vi "Editor.vi"(9 "Editor Events":T15, 11 "Printer Settings In":refnum<class "Printer Settings.lvclass">) -> (3 "Printer Settings Out":refnum<class "Printer Settings.lvclass">)   [LabVIEW 2023, in "VIDoc Printer.lvlib" / "Printer Settings.lvclass"]
uses:
  Printer Settings.lvclass
  Editors/VIDoc Editor/Editor Events Cluster.ctl
  Project Settings.ctl
  Interface Settings.ctl
  Detail Level Enum.ctl
  Scope Settings.ctl
  Class Settings.ctl
  Library Settings.ctl
  VI Settings.ctl
  Control Settings.ctl
  LLB Settings.ctl
  Formatting Options.ctl
  Background Formatting Cluster.ctl
  Bookmark Options.ctl
  Printer Settings.lvclass/Printer Settings.ctl
  Editors/VIDoc Editor/VIDocEditor.lvclass
panel:
  in  "Sections Tabs":T1(tab)
  in  "Format Options":T2={"Background"={"Public Scope"={"Option"=FALSE, "Color"=0, "Operator"=FALSE}, "Protected Scope"={"Option"=FALSE, "Color"=0, "Operator"=FALSE}, "Community Scope"={"Option"=FALSE, "Color"=0, "Operator"=FALSE}, "Private Scope"={"Option"=FALSE, "Color"=0, "Operator"=FALSE}, "Unknown Scope"={"Option"=FALSE, "Color"=0, "Operator"=FALSE}, "Auto Error Handling"={"Option"=FALSE, "Color"=0, "Operator"=FALSE}, "Inline"={"Option"=FALSE, "Color"=0, "Operator"=FALSE}, "Separate CC"={"Option"=FALSE, "Color"=0, "Operator"=FALSE}, "Execution Priority Normal"={"Option"=FALSE, "Color"=0, "Operator"=FALSE}, "Reentrancy Non-RE"={"Option"=FALSE, "Color"=0, "Operator"=FALSE}}, "Bookmark Options"={"Bookmarks as New Line in VI Descriptions"=TRUE, "Unique Bookmark Tags Only"=TRUE, "Include Tag and Text"=TRUE}}
  in  "Library Scope":T5={"Public"=TRUE, "Community"=TRUE, "Private"=TRUE, "Unknown"=TRUE}
  in  "Projects Enabled":bool=TRUE caption="Enabled"
  in  "Project":T6={"Paths"=TRUE, "Descriptions"=TRUE, "Memory"=TRUE, "Options"=TRUE, "Symbols"=TRUE}
  in  "Bookmark Term Settings":cluster{"Term":string, "Settings":T7}[](array[cluster])
  in  "Interface":T9={"Memory"=TRUE, "By List"=TRUE, "Details"=TRUE, "Detail Options"={"Description"=TRUE, "Properties"=TRUE, "Inheritance"=TRUE, "Inheritance Options"={"Parent Interfaces"=TRUE, "Friends"=TRUE}}, "List Detail Level"=enum."None", "Controls Detail Level"=enum."None", "Methods Detail Level"=enum."None", "Controls Scope"={"Public"=TRUE, "Protected"=TRUE, "Community"=TRUE, "Private"=TRUE, "Unknown"=TRUE}, "Methods Scope"={"Public"=TRUE, "Protected"=TRUE, "Community"=TRUE, "Private"=TRUE, "Unknown"=TRUE}}
  in  "Interfaces Enabled":bool=TRUE caption="Enabled"
  in  "Class":T11={"Memory"=TRUE, "By Folder"=TRUE, "By Tree"=TRUE, "By List"=TRUE, "Details"=TRUE, "Detail Options"={"Description"=TRUE, "Properties"=TRUE, "Inheritance"=TRUE, "Inheritance Options"={"Parent Classes"=TRUE, "Parent Interfaces"=TRUE, "Parent Libraries"=TRUE, "Friends"=TRUE}}, "CPD Detail Level"=enum."None", "List Detail Level"=enum."None", "Controls Detail Level"=enum."None", "Methods Detail Level"=enum."None", "Set Accessor Detail Level"=enum."None", "Get Accessor Detail Level"=enum."None", "Controls Scope"={"Public"=TRUE, "Protected"=TRUE, "Community"=TRUE, "Private"=TRUE, "Unknown"=TRUE}, "Methods Scope"={"Public"=TRUE, "Protected"=TRUE, "Community"=TRUE, "Private"=TRUE, "Unknown"=TRUE}, "Get Accessors Scope"={"Public"=TRUE, "Protected"=TRUE, "Community"=TRUE, "Private"=TRUE, "Unknown"=TRUE}, "Set Accessors Scope"={"Public"=TRUE, "Protected"=TRUE, "Community"=TRUE, "Private"=TRUE, "Unknown"=TRUE}}
  in  "Classes Enabled":bool=TRUE caption="Enabled"
  in  "Library":T12={"Memory"=TRUE, "By Folder"=TRUE, "By Tree"=TRUE, "By List"=TRUE, "Details"=TRUE, "Detail Options"={"Description"=TRUE, "Properties"=TRUE, "Friends"=TRUE, "Child Libraries"=TRUE}, "List Detail Level"=enum."None", "Methods Detail Level"=enum."None", "Controls Detail Level"=enum."None", "Methods Scope"={"Public"=TRUE, "Protected"=TRUE, "Community"=TRUE, "Private"=TRUE, "Unknown"=TRUE}, "Controls Scope"={"Public"=TRUE, "Protected"=TRUE, "Community"=TRUE, "Private"=TRUE, "Unknown"=TRUE}}
  in  "Libraries Enabled":bool=TRUE caption="Enabled"
  in  "VI Member":T7={"Memory"=TRUE, "By Folder"=TRUE, "By Tree"=TRUE, "By List"=TRUE, "Methods"=TRUE, "Method Options"={"Front Panels"=TRUE, "Options"=TRUE, "Controls"=TRUE}, "List Detail Level"=enum."None", "Methods Detail Level"=enum."None", "Controls Detail Level"=enum."None"}
  in  "VI Methods Enabled":bool=TRUE caption="Enabled"
  in  "Control Member":T13={"Memory"=TRUE, "By Folder"=TRUE, "By Tree"=TRUE, "By List"=TRUE, "Controls"=TRUE, "List Detail Level"=enum."None", "Controls Detail Level"=enum."None"}
  in  "Control Methods Enabled":bool=TRUE caption="Enabled"
  in  "LLB":T14={"Methods"=TRUE, "Controls"=TRUE, "Methods Detail Level"=enum."None", "Controls Detail Level"=enum."None"}
  in  "LLBs Enabled":bool=TRUE caption="Enabled"
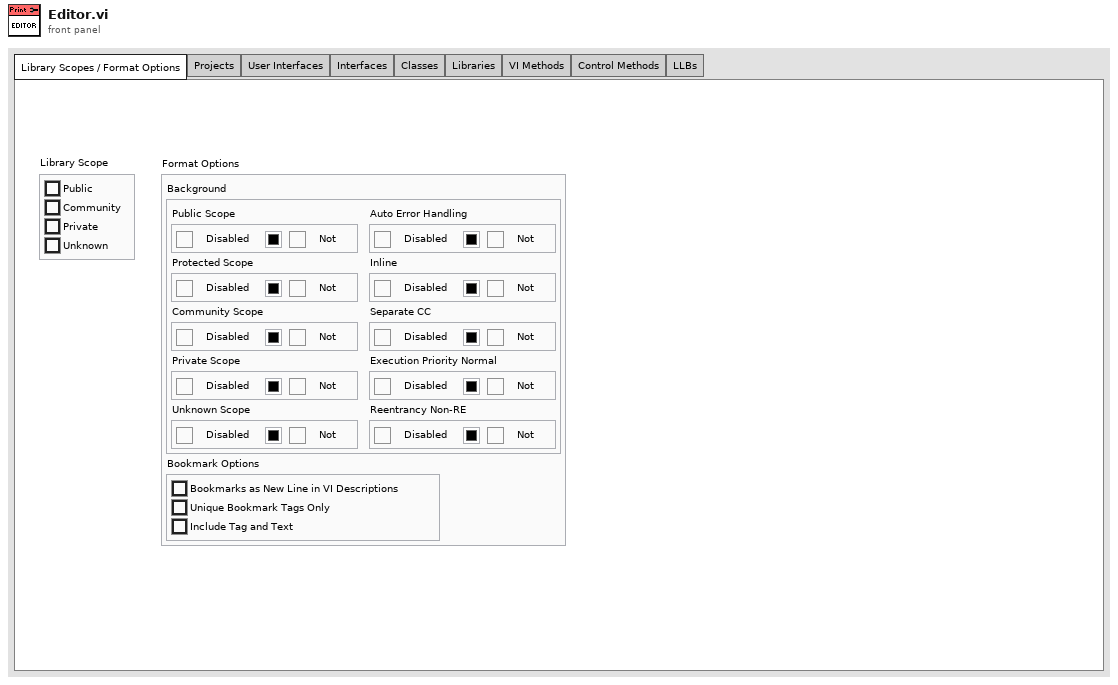
[diagram p1: front panel]
types:
  T1 = enum32{"Library Scopes / Format Options", "Projects", "User Interfaces", "Interfaces", "Classes", "Libraries", "VI Methods", "Control Methods", "LLBs"}
  T2 = typedef "VIDoc Printer.lvlib/Printer Settings.lvclass/Formatting Options.ctl" = cluster{"Background":cluster{"Public Scope":T3, "Protected Scope":T3, "Community Scope":T3, "Private Scope":T3, "Unknown Scope":T3, "Auto Error Handling":T3, "Inline":T3, "Separate CC":T3, "Execution Priority Normal":T3, "Reentrancy Non-RE":T3}, "Bookmark Options":T4}
  T3 = typedef "VIDoc Printer.lvlib/Printer Settings.lvclass/Background Formatting Cluster.ctl" = cluster{"Option":bool, "Color":u32, "Operator":bool}
  T4 = typedef "VIDoc Printer.lvlib/Printer Settings.lvclass/Bookmark Options.ctl" = cluster{"Bookmarks as New Line in VI Descriptions":bool, "Unique Bookmark Tags Only":bool, "Include Tag and Text":bool}
  T5 = cluster{"Public":bool, "Community":bool, "Private":bool, "Unknown":bool}
  T6 = typedef "VIDoc Printer.lvlib/Printer Settings.lvclass/Project Settings.ctl" = cluster{"Paths":bool, "Descriptions":bool, "Memory":bool, "Options":bool, "Symbols":bool}
  T7 = typedef "VIDoc Printer.lvlib/Printer Settings.lvclass/VI Settings.ctl" = cluster{"Memory":bool, "By Folder":bool, "By Tree":bool, "By List":bool, "Methods":bool, "Method Options":cluster{"Front Panels":bool, "Options":bool, "Controls":bool}, "List Detail Level":T8, "Methods Detail Level":T8, "Controls Detail Level":T8}
  T8 = typedef "VIDoc Printer.lvlib/Printer Settings.lvclass/Detail Level Enum.ctl" = enum16{"None", "Minimal", "Standard", "Full"}
  T9 = typedef "VIDoc Printer.lvlib/Printer Settings.lvclass/Interface Settings.ctl" = cluster{"Memory":bool, "By List":bool, "Details":bool, "Detail Options":cluster{"Description":bool, "Properties":bool, "Inheritance":bool, "Inheritance Options":cluster{"Parent Interfaces":bool, "Friends":bool}}, "List Detail Level":T8, "Controls Detail Level":T8, "Methods Detail Level":T8, "Controls Scope":T10, "Methods Scope":T10}
  T10 = typedef "VIDoc Printer.lvlib/Printer Settings.lvclass/Scope Settings.ctl" = cluster{"Public":bool, "Protected":bool, "Community":bool, "Private":bool, "Unknown":bool}
  T11 = typedef "VIDoc Printer.lvlib/Printer Settings.lvclass/Class Settings.ctl" = cluster{"Memory":bool, "By Folder":bool, "By Tree":bool, "By List":bool, "Details":bool, "Detail Options":cluster{"Description":bool, "Properties":bool, "Inheritance":bool, "Inheritance Options":cluster{"Parent Classes":bool, "Parent Interfaces":bool, "Parent Libraries":bool, "Friends":bool}}, "CPD Detail Level":T8, "List Detail Level":T8, "Controls Detail Level":T8, "Methods Detail Level":T8, "Set Accessor Detail Level":T8, "Get Accessor Detail Level":T8, "Controls Scope":T10, "Methods Scope":T10, "Get Accessors Scope":T10, "Set Accessors Scope":T10}
  T12 = typedef "VIDoc Printer.lvlib/Printer Settings.lvclass/Library Settings.ctl" = cluster{"Memory":bool, "By Folder":bool, "By Tree":bool, "By List":bool, "Details":bool, "Detail Options":cluster{"Description":bool, "Properties":bool, "Friends":bool, "Child Libraries":bool}, "List Detail Level":T8, "Methods Detail Level":T8, "Controls Detail Level":T8, "Methods Scope":T10, "Controls Scope":T10}
  T13 = typedef "VIDoc Printer.lvlib/Printer Settings.lvclass/Control Settings.ctl" = cluster{"Memory":bool, "By Folder":bool, "By Tree":bool, "By List":bool, "Controls":bool, "List Detail Level":T8, "Controls Detail Level":T8}
  T14 = typedef "VIDoc Printer.lvlib/Printer Settings.lvclass/LLB Settings.ctl" = cluster{"Methods":bool, "Controls":bool, "Methods Detail Level":T8, "Controls Detail Level":T8}
  T15 = typedef "VIDocEditor.lvclass/Editor Events Cluster.ctl" = cluster{"Close":refnum<user-event>, "Revert":refnum<user-event>, "Save":refnum<user-event>, "Changes?":refnum<user-event>}
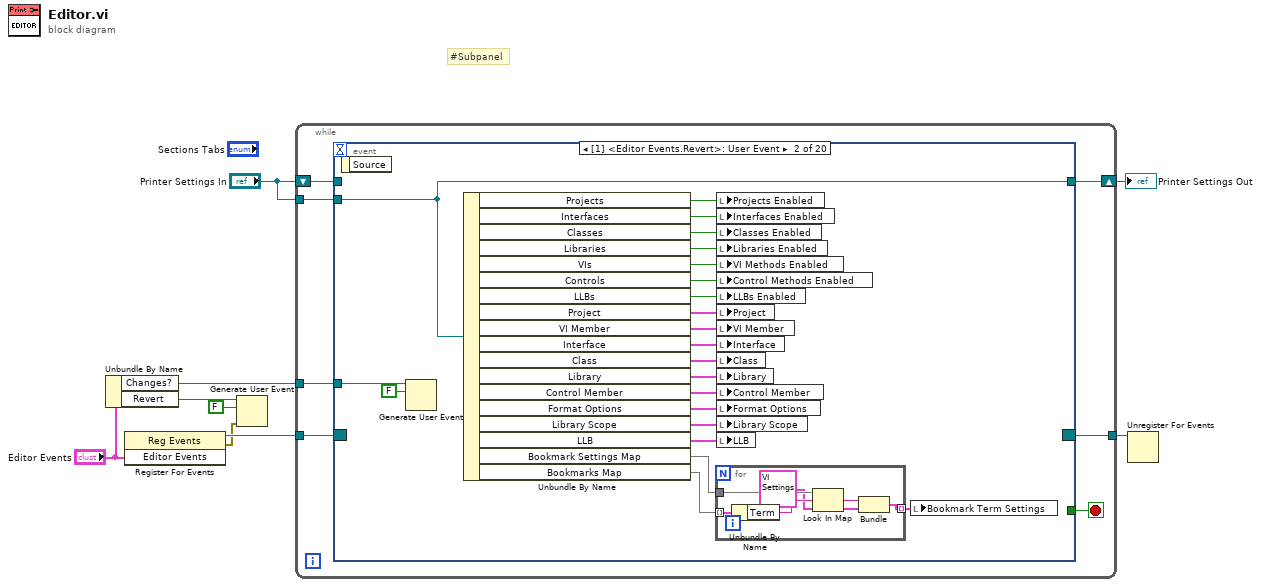
[diagram p0: block diagram]
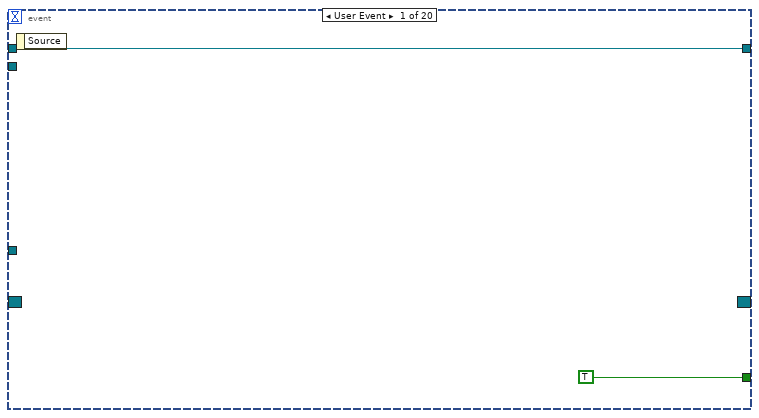
[diagram p2: hidden frame]
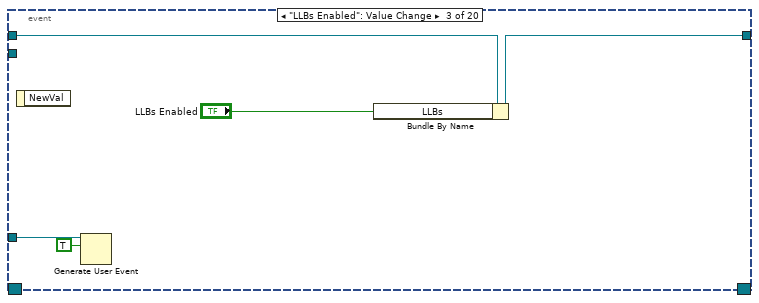
[diagram p3: hidden frame]
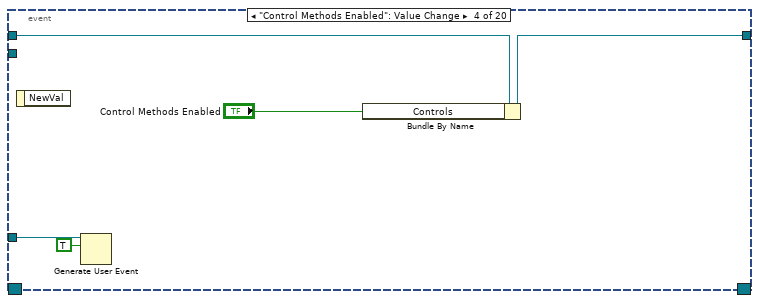
[diagram p4: hidden frame]
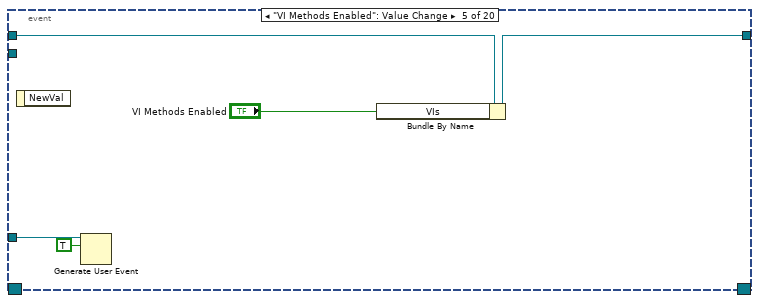
[diagram p5: hidden frame]
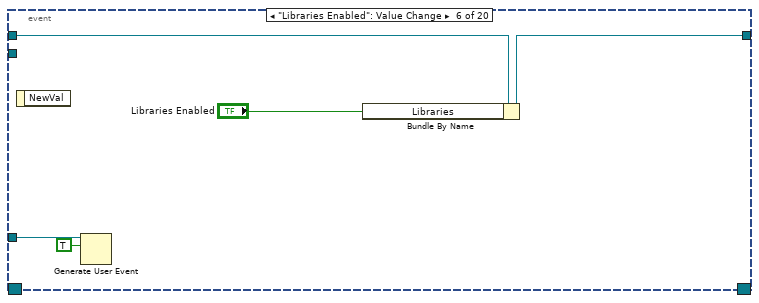
[diagram p6: hidden frame]
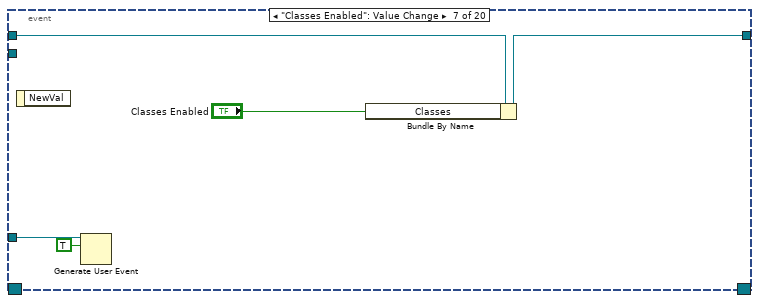
[diagram p7: hidden frame]
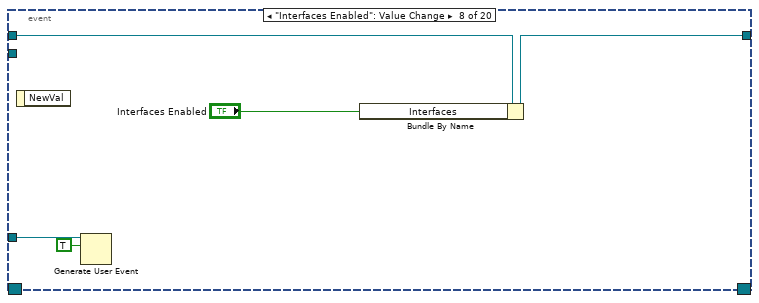
[diagram p8: hidden frame]
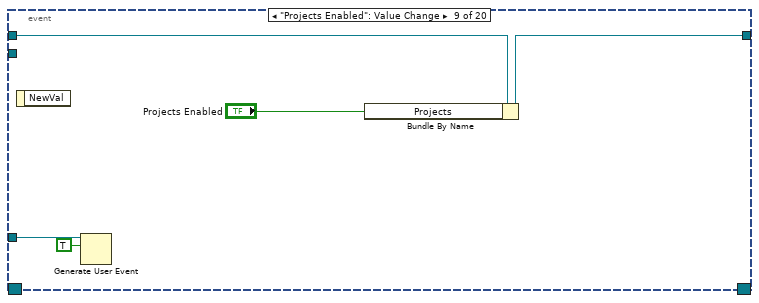
[diagram p9: hidden frame]
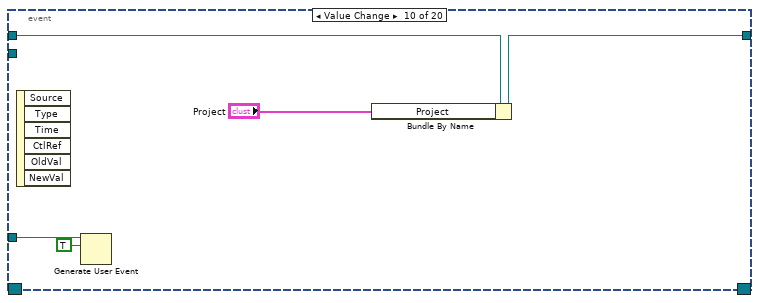
[diagram p10: hidden frame]
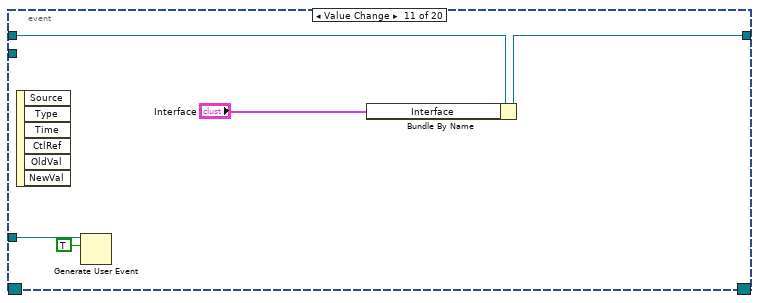
[diagram p11: hidden frame]
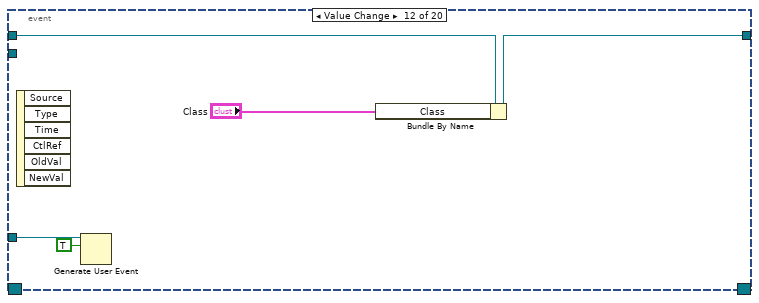
[diagram p12: hidden frame]
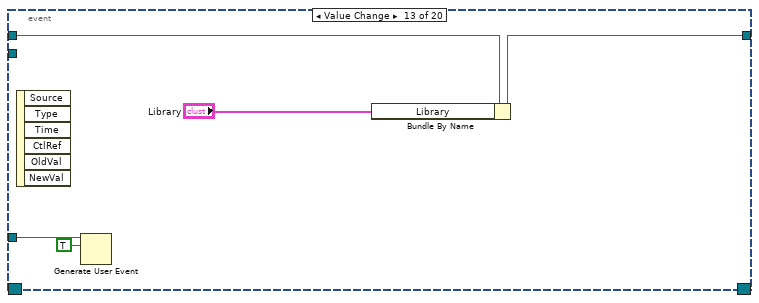
[diagram p13: hidden frame]
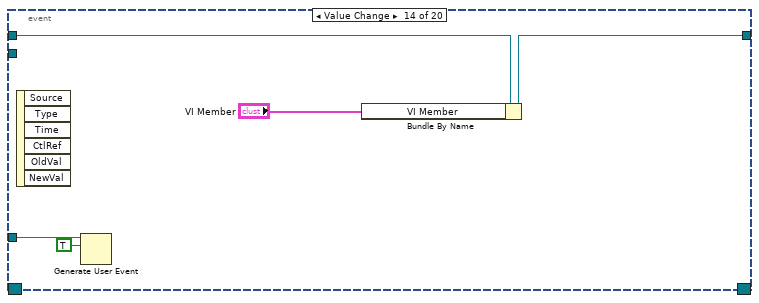
[diagram p14: hidden frame]
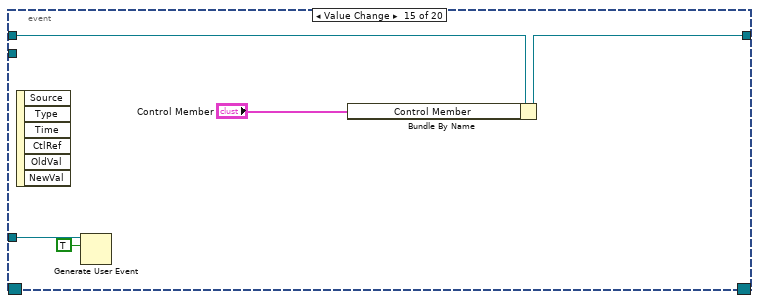
[diagram p15: hidden frame]
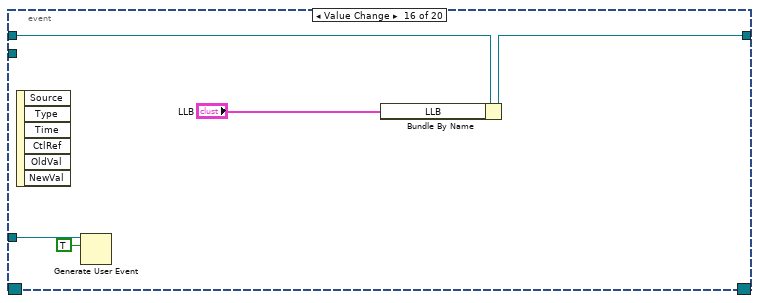
[diagram p16: hidden frame]
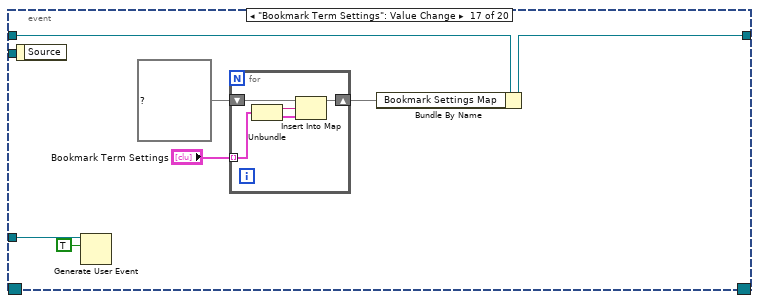
[diagram p17: hidden frame]
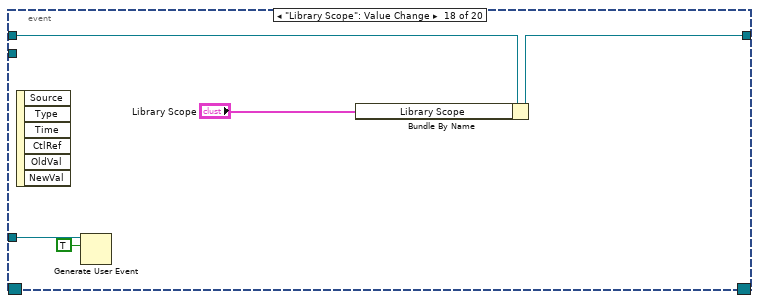
[diagram p18: hidden frame]
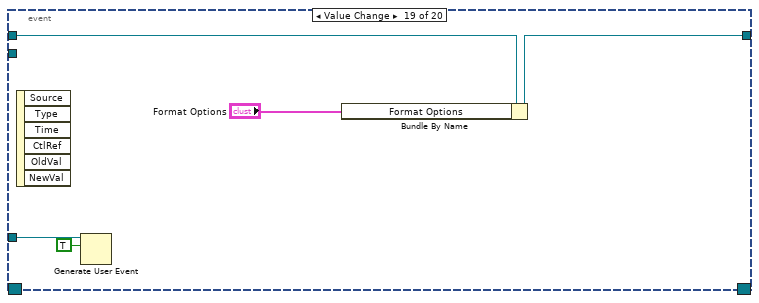
[diagram p19: hidden frame]
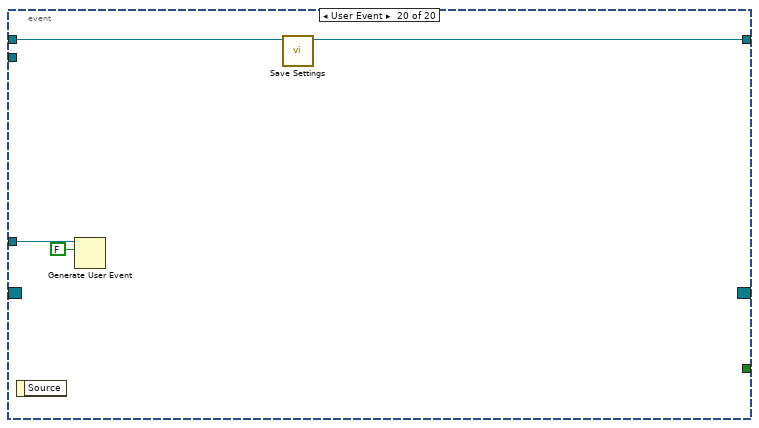
[diagram p20: hidden frame]
diagram:
  # "#Subpanel"
  n1 = Unbundle By Name("Editor Events") -> ("Changes?"=w1:refnum<user-event>, "Revert"=w4:refnum<user-event>)
  n2 = register-events("Editor Events") -> (reference out=w9:refnum<event-registration>, error out=w2:errorcluster)  [unwired: 2 in]
  n3 = Generate User Event(user event=w4, event data cluster=FALSE ("event data"), error in=w2) -> ()  [unwired: 1 in, 2 out]
  n4 = while {
    shift-right: [w14] -> w7
    shift-left: "Printer Settings In" -> [w16]
    tunnel: w9 -> [w15]
    tunnel: [w12] -> w8
    tunnel: "Printer Settings In" -> [w11]
    tunnel: w1 -> [w10]
    stop <- w13 stop-if-true
    n5 = event shown="[1] <Editor Events.Revert>: User Event" {
      selector: w15 -> [_ _ _ _ _ _ _ _ _ _ _ _ _ _ _ _ _ _ _ _]
      dyn-events: [_ _ _ _ _ _ _ _ _ _ _ _ _ _ _ _ _ _ _ _] -> w12
      timeout: _ -> [_ _ _ _ _ _ _ _ _ _ _ _ _ _ _ _ _ _ _ _]
      tunnel: w16 -> [w18 _ w51 w56 w61 w66 w71 w76 w81 w86 w91 w96 w101 w106 w111 w116 w123 w133 w138 w141]
      tunnel: [w18 w40 w50 w55 w60 w65 w70 w75 w80 w85 w90 w95 w100 w105 w110 w115 w122 w132 w137 w142] -> w14
      tunnel: [TRUE _ _ _ _ _ _ _ _ _ _ _ _ _ _ _ _ _ _ _] -> w13
      tunnel: w11 -> [_ w40 _ _ _ _ _ _ _ _ _ _ _ _ _ _ _ _ _ _]
      tunnel: w10 -> [_ w38 w47 w53 w58 w63 w68 w73 w78 w83 w88 w93 w98 w103 w108 w113 w120 w130 w135 w139]
      event User Event {
        n6 = event-data() -> ()  [unwired: 1 in, 1 out]
      }
      event User Event {
        n7 = event-data() -> ()  [unwired: 1 in, 1 out]
        n8 = Generate User Event(user event=w38, event data cluster=FALSE ("event data")) -> ()  [unwired: 2 in, 2 out]
        n9 = Unbundle By Name(w40) -> ("Projects"=w37:bool, "Interfaces"=w36:bool, "Classes"=w35:bool, "Libraries"=w34:bool, "VIs"=w33:bool, "Controls"=w32:bool, "LLBs"=w31:bool, "Project"=w29:T6, "VI Member"=w28:T7, "Interface"=w27:T9, "Class"=w26:T11, "Library"=w25:T12, "Control Member"=w24:T13, "Format Options"=w23:T2, "Library Scope"=w22:T5, "LLB"=w30:T14, "Bookmark Settings Map"=w20:map{string, T7}, "Bookmarks Map"=w21:map{string, string[]})
        n10 = for {
          tunnel: w21 -> [w46] mode=indexing
          tunnel: w20 -> [w45]
          tunnel: [w42] -> w19 mode=indexing
          n11 = Unbundle By Name(w46) -> ("Term"=w43:string)
          n12 = Look In Map(map=w45, key=w43, default value=T7 {"Memory"=FALSE, "By Folder"=FALSE, "By Tree"=TRUE, "By List"=FALSE, "Methods"=FALSE, "Method Options"={"Front Panels"=FALSE, "Options"=FALSE, "Controls"=FALSE}, "List Detail Level"=enum."Minimal", "Methods Detail Level"=enum."Minimal", "Controls Detail Level"=enum."Minimal"}) -> (value=w44:T7)  [unwired: 1 out]
          n13 = Bundle("Term"=w43, "Term Settings"=w44) -> (w42:cluster{"Term":string, "Term Settings":T7})  [unwired: 1 in]
        }
        n14 = local write "Projects Enabled"(w37) -> ()
        n15 = local write "Interfaces Enabled"(w36) -> ()
        n16 = local write "Classes Enabled"(w35) -> ()
        n17 = local write "Libraries Enabled"(w34) -> ()
        n18 = local write "VI Methods Enabled"(w33) -> ()
        n19 = local write "Control Methods Enabled"(w32) -> ()
        n20 = local write "LLBs Enabled"(w31) -> ()
        n21 = local write "Project"(w29) -> ()
        n22 = local write "VI Member"(w28) -> ()
        n23 = local write "Interface"(w27) -> ()
        n24 = local write "Class"(w26) -> ()
        n25 = local write "Library"(w25) -> ()
        n26 = local write "Control Member"(w24) -> ()
        n27 = local write "Format Options"(w23) -> ()
        n28 = local write "Library Scope"(w22) -> ()
        n29 = local write "LLB"(w30) -> ()
        n30 = local write "Bookmark Term Settings"(w19) -> ()
      }
      event "LLBs Enabled": Value Change {
        n31 = event-data() -> ()  [unwired: 1 in, 1 out]
        n32 = Generate User Event(user event=w47, event data cluster=TRUE ("event data")) -> ()  [unwired: 2 in, 2 out]
        n33 = Bundle By Name(cluster=w51, "LLBs"="LLBs Enabled") -> (w50:refnum<class "Printer Settings.lvclass">)
      }
      event "Control Methods Enabled": Value Change {
        n34 = event-data() -> ()  [unwired: 1 in, 1 out]
        n35 = Generate User Event(user event=w53, event data cluster=TRUE ("event data")) -> ()  [unwired: 2 in, 2 out]
        n36 = Bundle By Name(cluster=w56, "Controls"="Control Methods Enabled") -> (w55:refnum<class "Printer Settings.lvclass">)
      }
      event "VI Methods Enabled": Value Change {
        n37 = event-data() -> ()  [unwired: 1 in, 1 out]
        n38 = Generate User Event(user event=w58, event data cluster=TRUE ("event data")) -> ()  [unwired: 2 in, 2 out]
        n39 = Bundle By Name(cluster=w61, "VIs"="VI Methods Enabled") -> (w60:refnum<class "Printer Settings.lvclass">)
      }
      event "Libraries Enabled": Value Change {
        n40 = event-data() -> ()  [unwired: 1 in, 1 out]
        n41 = Generate User Event(user event=w63, event data cluster=TRUE ("event data")) -> ()  [unwired: 2 in, 2 out]
        n42 = Bundle By Name(cluster=w66, "Libraries"="Libraries Enabled") -> (w65:refnum<class "Printer Settings.lvclass">)
      }
      event "Classes Enabled": Value Change {
        n43 = event-data() -> ()  [unwired: 1 in, 1 out]
        n44 = Generate User Event(user event=w68, event data cluster=TRUE ("event data")) -> ()  [unwired: 2 in, 2 out]
        n45 = Bundle By Name(cluster=w71, "Classes"="Classes Enabled") -> (w70:refnum<class "Printer Settings.lvclass">)
      }
      event "Interfaces Enabled": Value Change {
        n46 = event-data() -> ()  [unwired: 1 in, 1 out]
        n47 = Generate User Event(user event=w73, event data cluster=TRUE ("event data")) -> ()  [unwired: 2 in, 2 out]
        n48 = Bundle By Name(cluster=w76, "Interfaces"="Interfaces Enabled") -> (w75:refnum<class "Printer Settings.lvclass">)
      }
      event "Projects Enabled": Value Change {
        n49 = event-data() -> ()  [unwired: 1 in, 1 out]
        n50 = Generate User Event(user event=w78, event data cluster=TRUE ("event data")) -> ()  [unwired: 2 in, 2 out]
        n51 = Bundle By Name(cluster=w81, "Projects"="Projects Enabled") -> (w80:refnum<class "Printer Settings.lvclass">)
      }
      event Value Change {
        n52 = event-data() -> ()  [unwired: 1 in, 6 out]
        n53 = Generate User Event(user event=w83, event data cluster=TRUE ("event data")) -> ()  [unwired: 2 in, 2 out]
        n54 = Bundle By Name(cluster=w86, "Project"="Project") -> (w85:refnum<class "Printer Settings.lvclass">)
      }
      event Value Change {
        n55 = event-data() -> ()  [unwired: 1 in, 6 out]
        n56 = Generate User Event(user event=w88, event data cluster=TRUE ("event data")) -> ()  [unwired: 2 in, 2 out]
        n57 = Bundle By Name(cluster=w91, "Interface"="Interface") -> (w90:refnum<class "Printer Settings.lvclass">)
      }
      event Value Change {
        n58 = event-data() -> ()  [unwired: 1 in, 6 out]
        n59 = Generate User Event(user event=w93, event data cluster=TRUE ("event data")) -> ()  [unwired: 2 in, 2 out]
        n60 = Bundle By Name(cluster=w96, "Class"="Class") -> (w95:refnum<class "Printer Settings.lvclass">)
      }
      event Value Change {
        n61 = event-data() -> ()  [unwired: 1 in, 6 out]
        n62 = Generate User Event(user event=w98, event data cluster=TRUE ("event data")) -> ()  [unwired: 2 in, 2 out]
        n63 = Bundle By Name(cluster=w101, "Library"="Library") -> (w100:refnum<class "Printer Settings.lvclass">)
      }
      event Value Change {
        n64 = event-data() -> ()  [unwired: 1 in, 6 out]
        n65 = Generate User Event(user event=w103, event data cluster=TRUE ("event data")) -> ()  [unwired: 2 in, 2 out]
        n66 = Bundle By Name(cluster=w106, "VI Member"="VI Member") -> (w105:refnum<class "Printer Settings.lvclass">)
      }
      event Value Change {
        n67 = event-data() -> ()  [unwired: 1 in, 6 out]
        n68 = Generate User Event(user event=w108, event data cluster=TRUE ("event data")) -> ()  [unwired: 2 in, 2 out]
        n69 = Bundle By Name(cluster=w111, "Control Member"="Control Member") -> (w110:refnum<class "Printer Settings.lvclass">)
      }
      event Value Change {
        n70 = event-data() -> ()  [unwired: 1 in, 6 out]
        n71 = Generate User Event(user event=w113, event data cluster=TRUE ("event data")) -> ()  [unwired: 2 in, 2 out]
        n72 = Bundle By Name(cluster=w116, "LLB"="LLB") -> (w115:refnum<class "Printer Settings.lvclass">)
      }
      event "Bookmark Term Settings": Value Change {
        n73 = event-data() -> ()  [unwired: 1 in, 1 out]
        n74 = Generate User Event(user event=w120, event data cluster=TRUE ("event data")) -> ()  [unwired: 2 in, 2 out]
        n75 = for {
          shift-right: [w127] -> w118
          shift-left: map{string, T7} {} ("Printer Settings.Bookmark Settings Map") -> [w128]
          tunnel: "Bookmark Term Settings" -> [w126] mode=indexing
          n76 = Unbundle(w126) -> ("Term"=w125:string, "Settings"=w124:T7)
          n77 = Insert Into Map(map in=w128, key=w125, value=w124) -> (map out=w127:map{string, T7})  [unwired: 2 out]
        }
        n78 = Bundle By Name(cluster=w123, "Bookmark Settings Map"=w118) -> (w122:refnum<class "Printer Settings.lvclass">)
      }
      event "Library Scope": Value Change {
        n79 = event-data() -> ()  [unwired: 1 in, 6 out]
        n80 = Generate User Event(user event=w130, event data cluster=TRUE ("event data")) -> ()  [unwired: 2 in, 2 out]
        n81 = Bundle By Name(cluster=w133, "Library Scope"="Library Scope") -> (w132:refnum<class "Printer Settings.lvclass">)
      }
      event Value Change {
        n82 = event-data() -> ()  [unwired: 1 in, 6 out]
        n83 = Generate User Event(user event=w135, event data cluster=TRUE ("event data")) -> ()  [unwired: 2 in, 2 out]
        n84 = Bundle By Name(cluster=w138, "Format Options"="Format Options") -> (w137:refnum<class "Printer Settings.lvclass">)
      }
      event User Event {
        n85 = event-data() -> ()  [unwired: 1 in, 1 out]
        n86 = Generate User Event(user event=w139, event data cluster=FALSE ("event data")) -> ()  [unwired: 2 in, 2 out]
        n87 = call-dynamic "Save Settings.vi"("Printer Settings In"=w141) -> ("Printer Settings Out"=w142:refnum<class "Printer Settings.lvclass">)  [unwired: 9 in, 1 out]
      }
    }
  }
  "Printer Settings Out" <- w7
  n88 = Unregister For Events(event registration refnum=w8) -> ()  [unwired: 1 in, 1 out]
